vi "Form Log Data String.vi"(8 "error in (no error)":errorcluster, 10 "Message Data In":variant, 11 "Log Text":string) -> (0 "error out":errorcluster, 3 "Log Data String":string)   [LabVIEW 2015, in "Generic Module Library.lvlib" / "Template G_Module.lvlib"]
uses:
  Template G_Module.lvlib
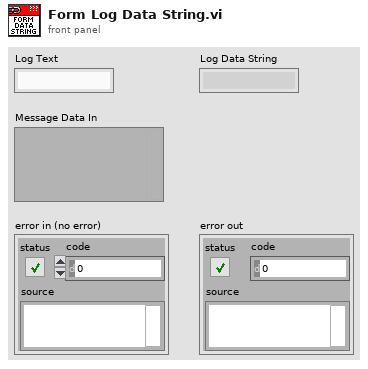
[diagram p1: front panel]
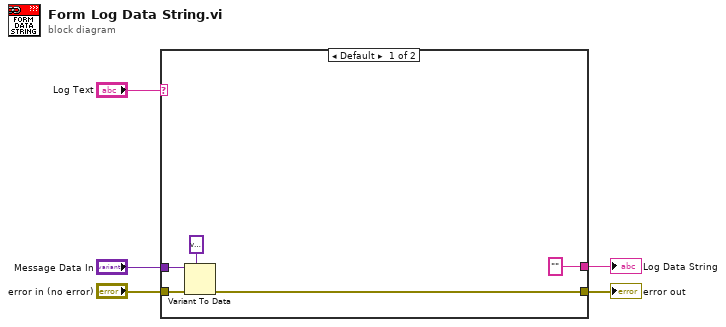
[diagram p0: block diagram]
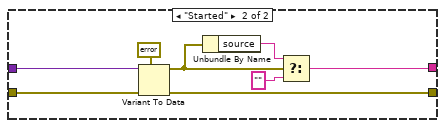
[diagram p2: hidden frame]
diagram:
  n1 = case shown="Default" "Log Text" {
    tunnel: "error in (no error)" -> [w10 w18]
    tunnel: [w9 w17] -> w1
    tunnel: "Message Data In" -> [w8 w16]
    tunnel: ["" w14] -> w4
    frame Default {
      n2 = Variant To Data(error in=w10, type=variant, Variant=w8) -> (error out=w9:errorcluster)  [unwired: 1 out]
    }
    frame "Started" {
      n3 = Variant To Data(error in=w18, type=errorcluster {"status"=FALSE, "code"=0, "source"=""} ("error in (no error)"), Variant=w16) -> (data=w12:errorcluster, error out=w17:errorcluster)
      n4 = Unbundle By Name(w12) -> ("source"=w11:string)
      n5 = Select(t=w11, s=w12, f="") -> (s? t:f=w14:string)
    }
  }
  "Log Data String" <- w4
  "error out" <- w1
